vi "CLD 10 Step Sequencer with CSV Front Panel.vi"() -> ()   [LabVIEW 2014]
doc: "CLD-Übung 10"
uses:
  CLD 10 CSV file read eum.ctl
  CLD 10 CSV file data structure.ctl
panel:
  out "Dauer des aktuellen Schritts":dbl
  out "Schritt 3":bool
  out "Schritt 2":bool
  out "Schritt 1":bool
  out "Zeit ist verstrichen":bool
  out "Verstrichene Zeit (s)":string
  in  "Autom. zurücksetzen":bool=TRUE
  in  "Zurücksetzen-Schaltfläche":bool
  in  "VI anhalten":bool
  out "Fehler (Ausgang)":errorcluster
  in  "Fehler (Eingang, kein Fehler)":errorcluster
  in  "Zielzeit (s)":dbl
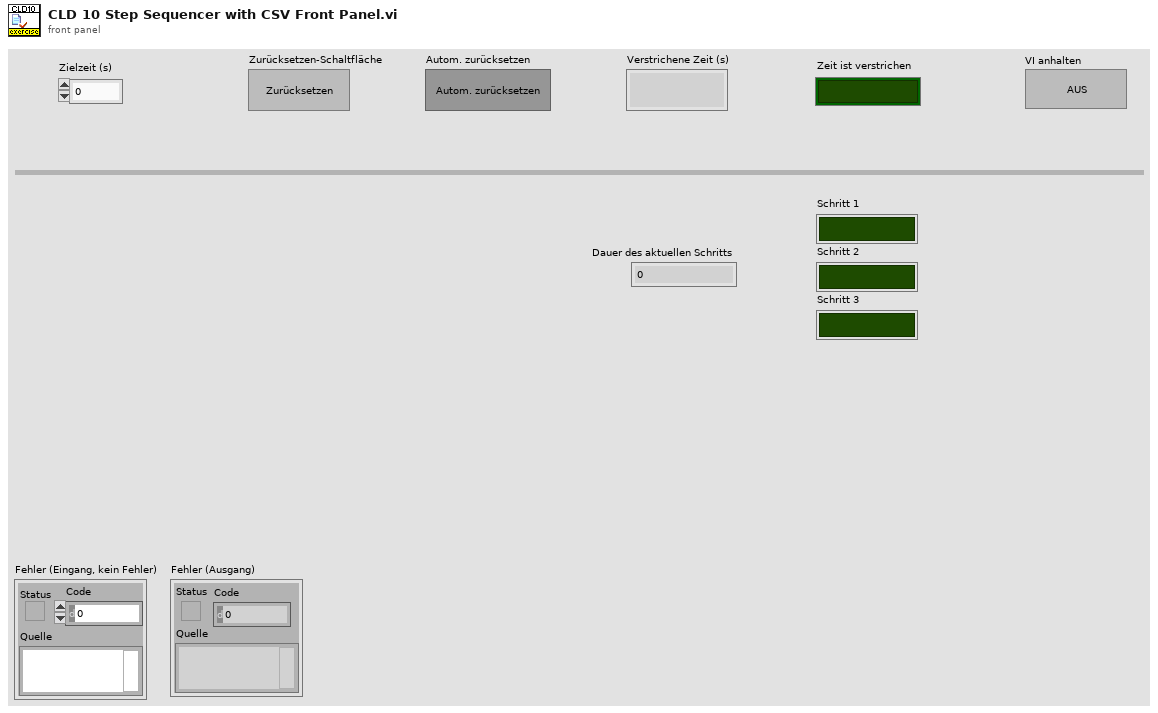
[diagram p1: front panel]
types:
  T1 = typedef "CLD 10 CSV file data structure.ctl" = cluster{"Schrittdauer - Ziel":i32, "Schritt 1":bool, "Schritt 2":bool, "Schritt 3":bool}
  T2 = typedef "CLD 10 CSV file read eum.ctl" = enum16{"CSV-Datei lesen", "Schritt eins ausführen", "Schritt zwei ausführen", "Schritt drei ausführen"}
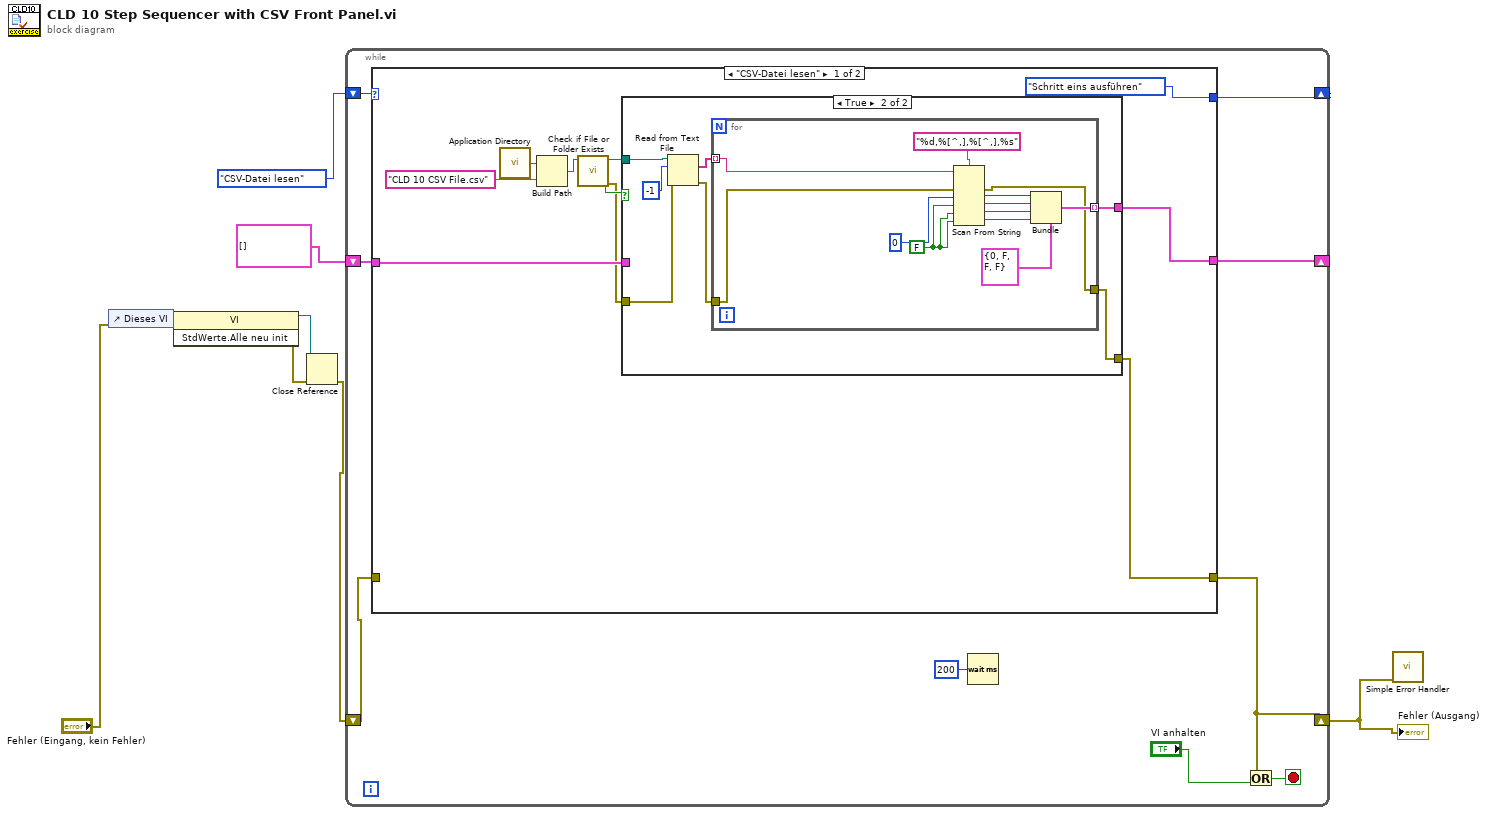
[diagram p0: block diagram]
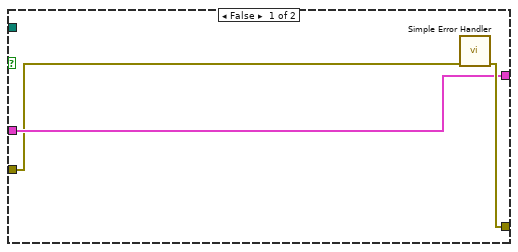
[diagram p2: hidden frame]
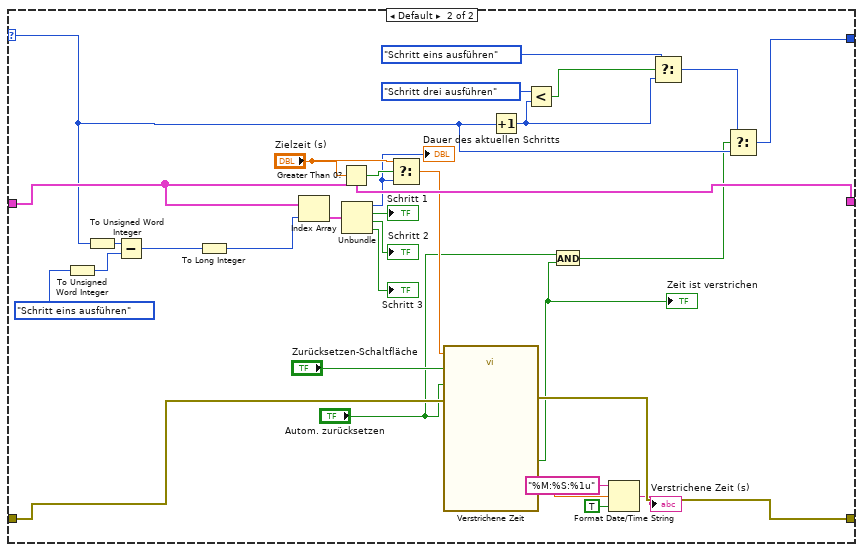
[diagram p3: hidden frame]
diagram:
  n1 = control-ref of="Dieses VI"() -> (w5:refnum<vi>)
  n2 = invoke class="VI" method="StdWerte.Alle neu init"(reference=w5, error in="Fehler (Eingang, kein Fehler)") -> (reference out=w4:refnum<vi>, error out=w3:errorcluster)  [unwired: 1 in, 1 out]
  n3 = Close Reference(reference=w4, error in (no error)=w3) -> (error out=w1:errorcluster)
  n4 = while {
    shift-right: [w10] -> _
    shift-left: CLD_10_CSV_file_read_eum."CSV-Datei lesen" ("CLD 10 - Timer-Enum") -> [w17]
    shift-right: [w11] -> _
    shift-left: T1[] [] -> [w16]
    shift-right: [w9] -> w6
    shift-left: w1 -> [w13]
    stop <- w15 stop-if-true
    n5 = case shown="\"CSV-Datei lesen\"" w17 {
      selector: w17 -> [_ w60]
      tunnel: [CLD_10_CSV_file_read_eum."Schritt eins ausführen" ("CLD 10 - Timer-Enum") w80] -> w10
      tunnel: w16 -> [w25 w79]
      tunnel: [w24 w79] -> w11
      tunnel: w13 -> [_ w78]
      tunnel: [w23 w77] -> w9
      frame "CSV-Datei lesen" {
        n6 = call <vilib>:"Application Directory.vi"() -> ("Application Directory"=w27:path)
        n7 = Build Path(base path=w27, name or relative path="CLD 10 CSV File.csv" ("Name oder relativer Pfad")) -> (appended path=w21:path)
        n8 = call <vilib>:"Check if File or Folder Exists.vi"("path"=w21) -> ("error out"=w18:errorcluster, "file or folder exists?"=w19:bool, "dup path"=w20:path)  [unwired: 8 in]
        n9 = case shown="True" w19 {
          tunnel: w25 -> [w29 _]
          tunnel: [w29 w37] -> w24
          tunnel: [w30 w36] -> w23
          tunnel: w20 -> [_ w34]
          tunnel: w18 -> [w28 w33]
          frame False {
            n10 = call <vilib>:"Simple Error Handler.vi"("error in (no error)"=w28) -> ("error out"=w30:errorcluster)  [unwired: 4 in, 4 out]
          }
          frame True {
            n11 = Read from Text File(file (use dialog)=w34, count=-1 ("Anzahl"), error in=w33) -> (text=w31:string[], error out=w32:errorcluster)  [unwired: 1 in, 2 out]
            n12 = for {
              tunnel: w32 -> [w38]
              tunnel: [w43] -> w37 mode=indexing
              tunnel: [w41] -> w36
              tunnel: w31 -> [w40] mode=indexing
              w49 = FALSE
              n13 = Scan From String(format string="%d,%[^,],%[^,],%s" ("Format-String"), input string=w40, error in=w38, default 1=0 ("Standardwert 1"), default 2=w49, default 3=w49, default 4=w49) -> (error out=w41:errorcluster, output 1=w48:i32, output 2=w47:bool, output 3=w46:bool, output 4=w45:bool)  [unwired: 1 in, 2 out]
              n14 = Bundle(cluster=T1 {"Schrittdauer - Ziel"=0, "Schritt 1"=FALSE, "Schritt 2"=FALSE, "Schritt 3"=FALSE} ("Datenstruktur der CSV-Datei"), "Schrittdauer - Ziel"=w48, "Schritt 1"=w47, "Schritt 2"=w46, "Schritt 3"=w45) -> (w43:T1)
            }
          }
        }
      }
      frame Default {
        n15 = To Unsigned Word Integer(number=CLD_10_CSV_file_read_eum."Schritt eins ausführen" ("y")) -> (unsigned 16bit integer=w56:u16)
        n16 = To Unsigned Word Integer(number=w60) -> (unsigned 16bit integer=w57:u16)
        n17 = Subtract(x=w57, y=w56) -> (x-y=w58:u16)
        n18 = To Long Integer(number=w58) -> (32bit integer=w55:i32)
        n19 = Index Array(array=w79, index=w55) -> (element=w76:T1)
        n20 = Greater Than 0?(x="Zielzeit (s)") -> (x > 0?=w69:bool)
        n21 = Unbundle(w76) -> ("Schrittdauer - Ziel"=w67:i32, "Schritt 1"=→"Schritt 1":bool, "Schritt 2"=→"Schritt 2":bool, "Schritt 3"=→"Schritt 3":bool)
        "Dauer des aktuellen Schritts" <- w67
        n22 = Select(t="Zielzeit (s)", s=w69, f=w67) -> (s? t:f=w66:dbl)
        n23 = call "Verstrichene Zeit"("Time Target (s)"=w66, "Reset"="Zurücksetzen-Schaltfläche", "Auto Reset"="Autom. zurücksetzen", "error in (no error)"=w78) -> ("Elapsed Time (s)"=w71:dbl, "Time has Elapsed"=w52:bool, "error out"=w77:errorcluster)  [unwired: 8 in, 5 out]
        "Zeit ist verstrichen" <- w52
        n24 = Increment(x=w60) -> (x+1=w53:T2)
        n25 = Less?(x=CLD_10_CSV_file_read_eum."Schritt drei ausführen", y=w53) -> (x < y?=w62:bool)
        n26 = And(x="Autom. zurücksetzen", y=w52) -> (x .and. y?=w50:bool)
        n27 = Format Date/Time String(time format string (%c)="%M:%S:%1u" ("Zeitformatierungs-String (%c)"), seconds (now)=w71, UTC format=TRUE ("Angabe von Sekunden? (F)")) -> (date/time string=→"Verstrichene Zeit (s)":string)
        n28 = Select(t=CLD_10_CSV_file_read_eum."Schritt eins ausführen" ("x"), s=w62, f=w53) -> (s? t:f=w61:T2)
        n29 = Select(t=w61, s=w50, f=w60) -> (s? t:f=w80:T2)
      }
    }
    n30 = Wait (ms)(milliseconds to wait=u32 200 ("Zu wartende ms")) -> ()  [unwired: 1 out]
    n31 = Or(x=w9, y="VI anhalten") -> (x .or. y?=w15:bool)
  }
  "Fehler (Ausgang)" <- w6
  n32 = call <vilib>:"Simple Error Handler.vi"("error in (no error)"=w6) -> ()  [unwired: 4 in, 5 out]
